vi "(SubVI) POS_of_cards.vi"() -> (0 "POS_of_cards":T1[](array[typedef]))   [LabVIEW 2018]
uses:
  <vilib>/Utility/miscctls.llb/LVPositionTypeDef.ctl
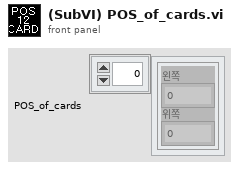
[diagram p1: front panel]
types:
  T1 = typedef "LVPositionTypeDef.ctl" = cluster{"Left":i32, "Top":i32}
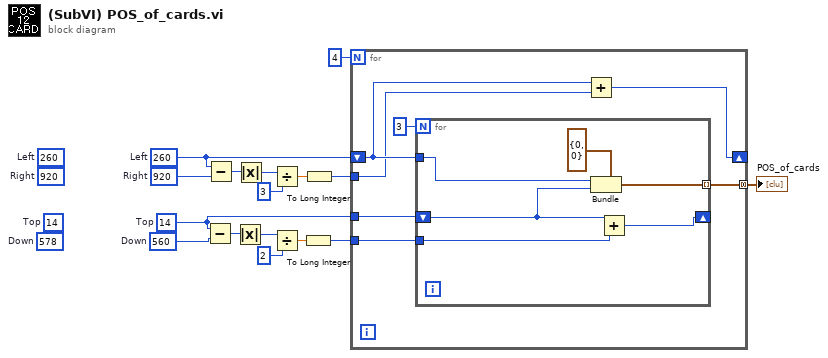
[diagram p0: block diagram]
diagram:
  (unwired) 920  # Right
  (unwired) 260  # Left
  (unwired) 578  # Down
  (unwired) 14  # Top
  w3 = 920  # Right
  w10 = 260  # Left
  w2 = 560  # Down
  w12 = 14  # Top
  n1 = Subtract(x=w12, y=w2) -> (x-y=w4:i32)
  n2 = Subtract(x=w10, y=w3) -> (x-y=w5:i32)
  n3 = Absolute Value(x=w4) -> (abs(x)=w9:i32)
  n4 = Absolute Value(x=w5) -> (abs(x)=w6:i32)
  n5 = Divide(x=w6, y=3) -> (x/y=w14:dbl)
  n6 = Divide(x=w9, y=2) -> (x/y=w13:dbl)
  n7 = To Long Integer(number=w13) -> (32bit integer=w16:i32)
  n8 = To Long Integer(number=w14) -> (32bit integer=w15:i32)
  n9 = for {
    N: 4 -> [_]
    shift-right: [w18] -> _
    shift-left: w10 -> [w20]
    tunnel: w12 -> [w22]
    tunnel: w15 -> [w19]
    tunnel: w16 -> [w21]
    tunnel: [w17] -> w1 mode=concatenating
    n10 = for {
      N: 3 -> [_]
      shift-right: [w28] -> _
      shift-left: w22 -> [w26]
      tunnel: w20 -> [w27]
      tunnel: w21 -> [w29]
      tunnel: [w24] -> w17 mode=indexing
      n11 = Bundle(cluster=T1 {"Left"=0, "Top"=0} ("위치"), "Left"=w27, "Top"=w26) -> (w24:T1)
      n12 = Add(x=w26, y=w29) -> (x+y=w28:i32)
    }
    n13 = Add(x=w20, y=w19) -> (x+y=w18:i32)
  }
  "POS_of_cards" <- w1
